vi "SVD-1D.vi"(5 "Data in":cdb[](array[numeric])) -> (3 "G2":dbl[](array[numeric]), 4 "Singular Values":dbl[](graph), 6 "Matrix U":T2, 8 "Matrix S":T2, 10 "Matrix V":T2, 13 "GapCutOff":i16, 14 "Hs":cdb[][](array[numeric]), 15 "SV Gap Ratio":dbl[](array[numeric]))   [LabVIEW 2022 SP3]
uses:
  <vilib>/Analysis/Matrix/Datatypes/RealMatrix.ctl
  <vilib>/Analysis/Matrix/Datatypes/ComplexMatrix.ctl
  <vilib>/Analysis/7linalg.llb/Complex SVD Decomposition.vi
  <vilib>/Analysis/NI_AALPro.lvlib
  <vilib>/Analysis/Matrix/NI_Matrix.lvlib
panel:
  out "Matrix V 2":T1
  out "Matrix S 2":T1
  out "Matrix U 2":T1
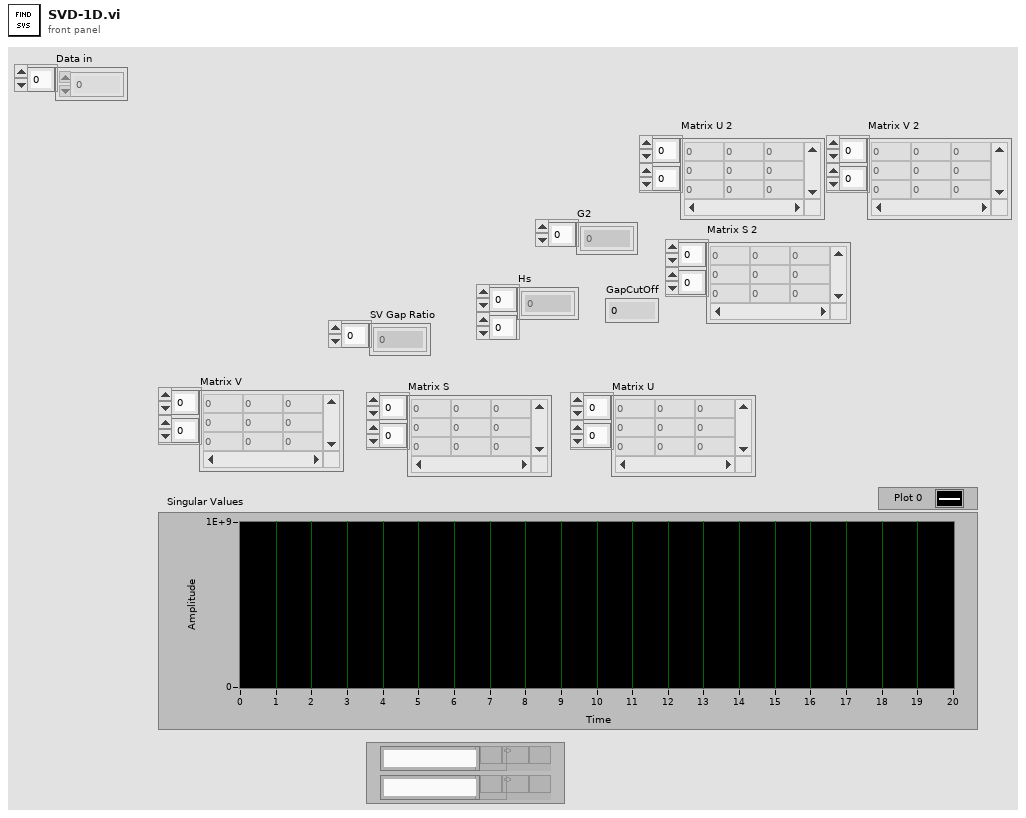
[diagram p1: front panel]
types:
  T1 = typedef "NI_Matrix.lvlib/ComplexMatrix.ctl" = cdb[][]
  T2 = typedef "NI_Matrix.lvlib/RealMatrix.ctl" = dbl[][]
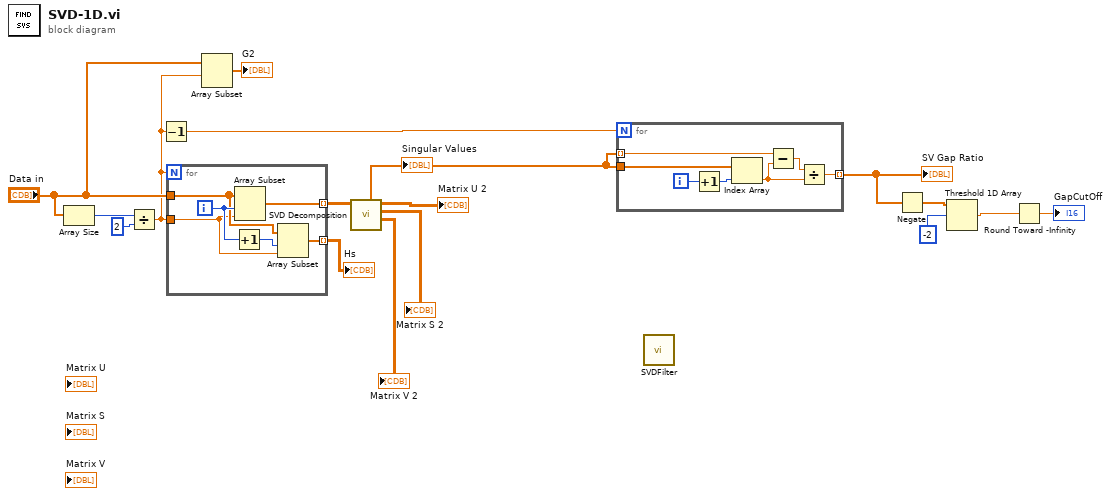
[diagram p0: block diagram]
diagram:
  n1 = Array Size(array="Data in") -> (size(s)=w17:i32)
  n2 = Divide(x=w17, y=2) -> (x/y=w10:dbl)
  n3 = Decrement(x=w10) -> (x-1=w13:dbl)
  n4 = for {
    N: w10 -> [_]
    tunnel: w10 -> [w19]
    tunnel: [w23] -> w16 mode=indexing
    tunnel: "Data in" -> [w20]
    tunnel: [w18] -> w15 mode=indexing
    i -> [w22]
    n5 = Increment(x=w22) -> (x+1=w21:i32)
    n6 = Array Subset(array=w20, index=w22, length=w19) -> (w23:cdb[])
    n7 = Array Subset(array=w20, index=w21, length=w19) -> (w18:cdb[])
  }
  "Hs" <- w15
  n8 = Array Subset(array="Data in", index=w10) -> (→"G2":cdb[])  [unwired: 1 in]
  n9 = call-poly <vilib>:"SVD Decomposition.vi"("A"=w16) -> ("Matrix V"=→"Matrix V 2":T1, "Matrix S"=→"Matrix S 2":T1, "Matrix U"=→"Matrix U 2":T1, "Vector S"=w12:dbl[])  [unwired: 6 in, 1 out]
  "Singular Values" <- w12
  n10 = for {
    N: w13 -> [_]
    tunnel: w12 -> [w29]
    tunnel: w12 -> [w25] mode=indexing
    tunnel: [w26] -> w8 mode=indexing
    i -> [w30]
    n11 = Increment(x=w30) -> (x+1=w27:i32)
    n12 = Index Array(array=w29, index=w27) -> (element=w24:dbl)
    n13 = Subtract(x=w25, y=w24) -> (x-y=w28:dbl)
    n14 = Divide(x=w28, y=w24) -> (x/y=w26:dbl)
  }
  "SV Gap Ratio" <- w8
  n15 = call "SVDFilter.vi"() -> ()  [unwired: 10 in, 2 out]
  n16 = Negate(x=w8) -> (-x=w7:dbl[])
  n17 = Threshold 1D Array(2:-2, 3:w7) -> (0:w5:dbl)  [unwired: 1 in]
  n18 = Round Toward -Infinity(1:w5) -> (0:→"GapCutOff":dbl)
